vi "Sequence.CreateCase.vi"(6 "Skip":T1, 7 "Iteration":string, 8 "error in (no error)":errorcluster, 9 "Condition":T2, 10 "Refs":T4, 11 "TaskRef":refnum<k24>) -> (0 "error out":errorcluster)   [LabVIEW 2015, in "Single Station Execution.lvlib"]
uses:
  Single Station Execution.lvlib
  NationalInstruments.VeriStand.RealTimeSequenceDefinitionApi
  Types/Sequence.MainSeqRefs.ctl
  Types/Conditions.OperationTypes.ctl
  Types/Compiled.StepCondition.ctl
  Types/Channel.Properties.ctl
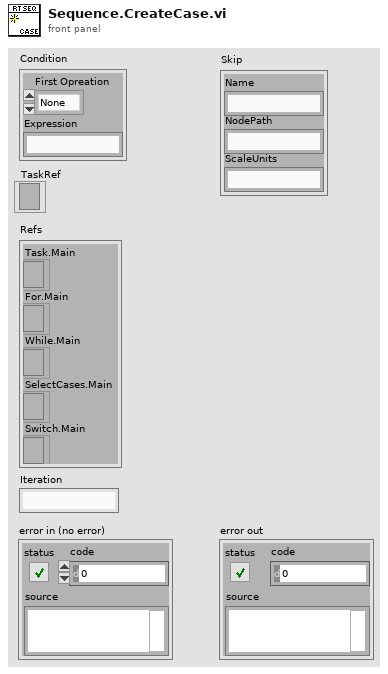
[diagram p1: front panel]
types:
  T1 = typedef "Single Station Execution.lvlib/Channel.Properties.ctl" = cluster{"Name":string, "NodePath":string, "ScaleUnits":string}
  T2 = typedef "Single Station Execution.lvlib/Compiled.StepCondition.ctl" = cluster{"First Opreation":T3, "Expression":string}
  T3 = typedef "Single Station Execution.lvlib/Conditions.OperationTypes.ctl" = enum8{"None", "&&", "||"}
  T4 = typedef "Single Station Execution.lvlib/Sequence.MainSeqRefs.ctl" = cluster{"Task.Main":refnum<k24>, "For.Main":refnum<k24>, "While.Main":refnum<k24>, "SelectCases.Main":refnum<k24>, "Switch.Main":refnum<k24>}
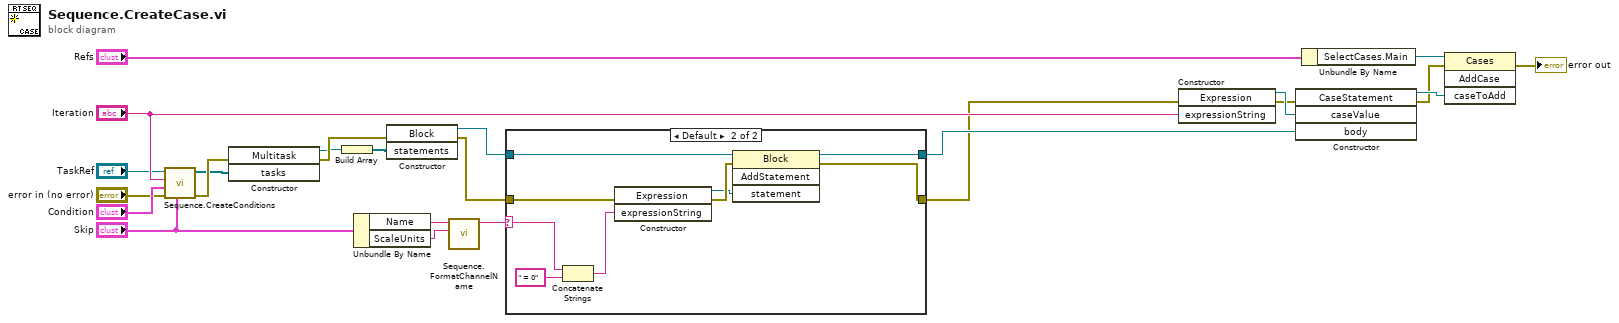
[diagram p0: block diagram]
diagram:
  n1 = call "Sequence.CreateConditions.vi"("Skip"="Skip", "error in (no error)"="error in (no error)", "Condition"="Condition", "Iteration"="Iteration", "Task"="TaskRef") -> ("error out"=w21:errorcluster, "Tasks"=w20:refnum<k24>[])  [unwired: 5 in]
  n2 = constructor class="Multitask"(error in=w21, "tasks"=w20) -> (reference out=w18:refnum<k24>, error out=w19:errorcluster)  [unwired: 2 in, 2 out]
  n3 = Build Array(w18) -> (w17:refnum<k24>[])
  n4 = Unbundle By Name("Skip") -> ("Name"=w6:string, "ScaleUnits"=w7:string)
  n5 = constructor class="Block"(error in=w19, "statements"=w17) -> (reference out=w5:refnum<k24>, error out=w3:errorcluster)  [unwired: 2 in, 2 out]
  n6 = call "Sequence.FormatChannelName.vi"("ScaleUnits"=w7, "Name"=w6) -> ("ChannelName"=w8:string)  [unwired: 9 in]
  n7 = case shown="Default" w8 {
    selector: w8 -> [_ w32]
    tunnel: [w26 w30] -> w2
    tunnel: w5 -> [w25 w31]
    tunnel: w3 -> [w26 w33]
    tunnel: [w25 w29] -> w4
    frame "" {
    }
    frame Default {
      n8 = Concatenate Strings(w32, " = 0" ("string")) -> (w34:string)
      n9 = constructor class="Expression"(error in=w33, "expressionString"=w34) -> (reference out=w27:refnum<k24>, error out=w28:errorcluster)  [unwired: 2 in, 2 out]
      n10 = invoke class="Block" method="AddStatement"(reference=w31, error in=w28, "statement"=w27) -> (reference out=w29:refnum<k24>, error out=w30:errorcluster)  [unwired: 1 in, 2 out]
    }
  }
  n11 = constructor class="Expression"(error in=w2, "expressionString"="Iteration") -> (reference out=w16:refnum<k24>, error out=w12:errorcluster)  [unwired: 2 in, 2 out]
  n12 = constructor class="CaseStatement"(error in=w12, "caseValue"=w16, "body"=w4) -> (reference out=w14:refnum<k24>, error out=w13:errorcluster)  [unwired: 2 in, 3 out]
  n13 = Unbundle By Name("Refs") -> ("SelectCases.Main"=w24:refnum<k24>)
  n14 = invoke class="Cases" method="AddCase"(reference=w24, error in=w13, "caseToAdd"=w14) -> (error out=→"error out":errorcluster)  [unwired: 1 in, 3 out]
